vi "Parameter Channel to Strings.vi"(11 "parameter channel definition":T3={"name"="", "default value"=1.0, "unit"="", "parameter definition"={"start index"=0, "size (bits)"=16, "encoding"=enum."BNR", "signed"=TRUE, "multiplier"=1.0, "offset"=0.0}}) -> (3 "parameter channel strings":T1, 5 "name strings":T1)   [LabVIEW 2020, in "Ballard MIL-STD-1553 System Explorer.lvlib" / "Implementation.lvlib" / "Refresh.lvlib"]
uses:
  Refresh.lvlib
  Shared/Parameter Definition.ctl
  Scripting/Constants.vi
  Scripting/Ballard MIL-STD-1553 Scripting.lvlib
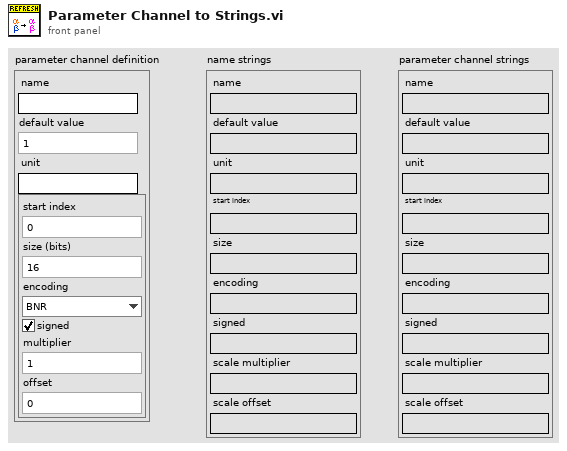
[diagram p1: front panel]
types:
  T1 = cluster{"name":string, "default value":string, "unit":string, "start index":string, "size":string, "encoding":string, "signed":string, "scale multiplier":string, "scale offset":string}
  T2 = typedef "Parameter Definition.ctl" = cluster{"start index":i32, "size (bits)":i32, "encoding":enum16{"BNR", "BCD", "Discrete"}, "signed":bool, "multiplier":dbl, "offset":dbl}
  T3 = cluster{"name":string, "default value":dbl, "unit":string, "parameter definition":T2}
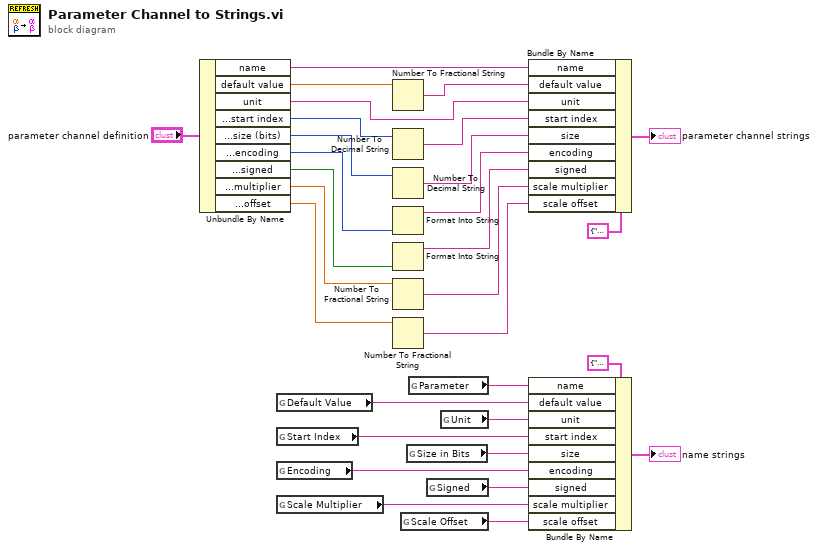
[diagram p0: block diagram]
diagram:
  n1 = Unbundle By Name("parameter channel definition") -> ("name"=w30:string, "default value"=w29:dbl, "unit"=w27:string, "parameter definition.start index"=w26:i32, "parameter definition.size (bits)"=w25:i32, "parameter definition.encoding"=w22:enum16{"BNR", "BCD", "Discrete"}, "parameter definition.signed"=w15:bool, "parameter definition.multiplier"=w21:dbl, "parameter definition.offset"=w20:dbl)
  n2 = global read "Constants.vi" "Default Value"() -> (w9:string)
  n3 = global read "Constants.vi" "Start Index"() -> (w7:string)
  n4 = global read "Constants.vi" "Encoding"() -> (w5:string)
  n5 = global read "Constants.vi" "Scale Multiplier"() -> (w3:string)
  n6 = Number To Fractional String(number=w29) -> (F-format string=w28:string)  [unwired: 3 in]
  n7 = Number To Decimal String(number=w26) -> (decimal integer string=w24:string)  [unwired: 1 in]
  n8 = Number To Decimal String(number=w25) -> (decimal integer string=w23:string)  [unwired: 1 in]
  n9 = Format Into String(w22) -> (resulting string=w17:string)  [unwired: 3 in, 1 out]
  n10 = Format Into String(w15) -> (resulting string=w16:string)  [unwired: 3 in, 1 out]
  n11 = Number To Fractional String(number=w21) -> (F-format string=w19:string)  [unwired: 3 in]
  n12 = Number To Fractional String(number=w20) -> (F-format string=w18:string)  [unwired: 3 in]
  n13 = global read "Constants.vi" "Scale Offset"() -> (w2:string)
  n14 = global read "Constants.vi" "Size in Bits"() -> (w6:string)
  n15 = global read "Constants.vi" "Parameter"() -> (w10:string)
  n16 = global read "Constants.vi" "Signed"() -> (w4:string)
  n17 = global read "Constants.vi" "Unit"() -> (w8:string)
  n18 = Bundle By Name(cluster=T1 {"name"="", "default value"="", "unit"="", "start index"="", "size"="", "encoding"="", "signed"="", "scale multiplier"="", "scale offset"=""} ("parameter channel strings"), "name"=w30, "default value"=w28, "unit"=w27, "start index"=w24, "size"=w23, "encoding"=w17, "signed"=w16, "scale multiplier"=w19, "scale offset"=w18) -> (→"parameter channel strings":T1)
  n19 = Bundle By Name(cluster=T1 {"name"="", "default value"="", "unit"="", "start index"="", "size"="", "encoding"="", "signed"="", "scale multiplier"="", "scale offset"=""} ("name strings"), "name"=w10, "default value"=w9, "unit"=w8, "start index"=w7, "size"=w6, "encoding"=w5, "signed"=w4, "scale multiplier"=w3, "scale offset"=w2) -> (→"name strings":T1)
